vi "Gainadjustmentch0.vi"(1 "Gain":dbl[](array[numeric])=[100.0, 100.0, 100.0, 100.0, 100.0, 100.0, 100.0, 100.0, 100.0, 100.0, 100.0, 100.0, 100.0, 100.0, 100.0, 100.0, 100.0, 100.0, 100.0, 100.0, 100.0, 100.0, 100.0, 100.0, 100.0, 100.0, 100.0, 100.0, 100.0, 100.0, 100.0]) -> (0 "Adjusted gain":dbl[](array[numeric])=[99.5, 99.5, 99.5, 99.5, 99.5, 99.5, 99.5, 99.5, 99.5, 99.5, 99.5, 99.5, 99.5, 99.5, 99.5, 99.5, 99.5, 99.5, 99.5, 99.5, 99.5, 99.5, 99.5, 99.5, 99.5, 99.5, 99.5, 99.5, 99.5, 99.5, 99.5])   [LabVIEW 2020]
uses:
  <vilib>/Utility/file.llb/Read From Spreadsheet File (DBL).vi
  <vilib>/gmath/NI_Gmath.lvlib
panel:
  in  "CH 0 Data Path (.csv)":path=path "C:/Users/yalem/Documents/Optlev/LabView Code/ARRAY/Power Normalization Files/10-13ch0gainvpower.csv"
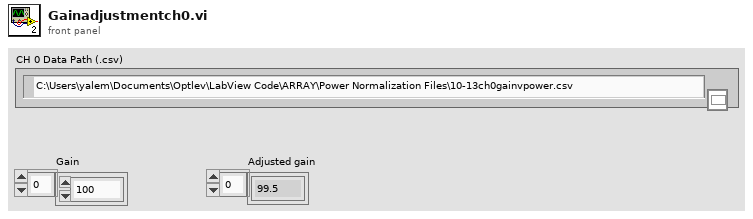
[diagram p1: front panel]
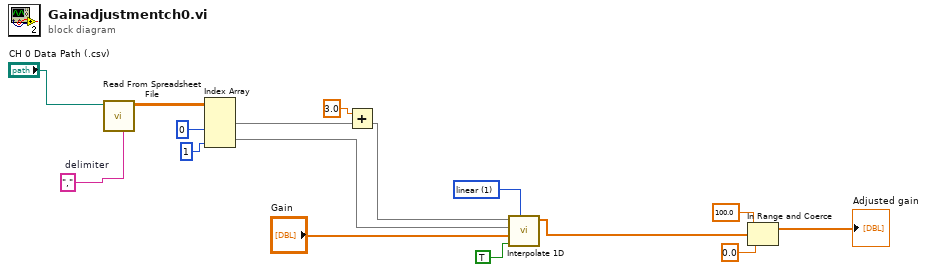
[diagram p0: block diagram]
diagram:
  w12 = 1 items=["nearest", "linear", "spline", "cubic Hermite", "Lagrange"] ("method")
  w15 = ","  # delimiter
  n1 = call-poly <vilib>:"Read From Spreadsheet File.vi"("delimiter (\\t)"=w15, "file path (dialog if empty)"="CH 0 Data Path (.csv)") -> ("all rows"=w14:dbl[][])  [unwired: 5 in, 4 out]
  n2 = Index Array(array=w14, index (col) #1=0, index (col) #2=1) -> (element #1=w2:dbl[], element #2=w4:dbl[])  [unwired: 2 in]
  n3 = Add(x=3.0, y=w2) -> (x+y=w3:dbl[])
  n4 = call <vilib>:"Interpolate 1D.vi"("method"=w12, "X is monotonic"=TRUE, "xi"="Gain", "X"=w4, "Y"=w3) -> ("yi"=w10:dbl[])  [unwired: 4 in, 2 out]
  n5 = In Range and Coerce(upper limit=100.0, x=w10, lower limit=0.0) -> (coerced(x)=→"Adjusted gain":dbl[])  [unwired: 1 out]
